vi "StudentDataBase.vi"() -> ()   [LabVIEW 2020]
uses:
  #typedef_Student.ctl
panel:
  out "Repeated students by name":T1[](array[typedef])
  out "Sorted students by number":T1[](array[typedef])
  in  "List of Students":T1[](array[typedef])
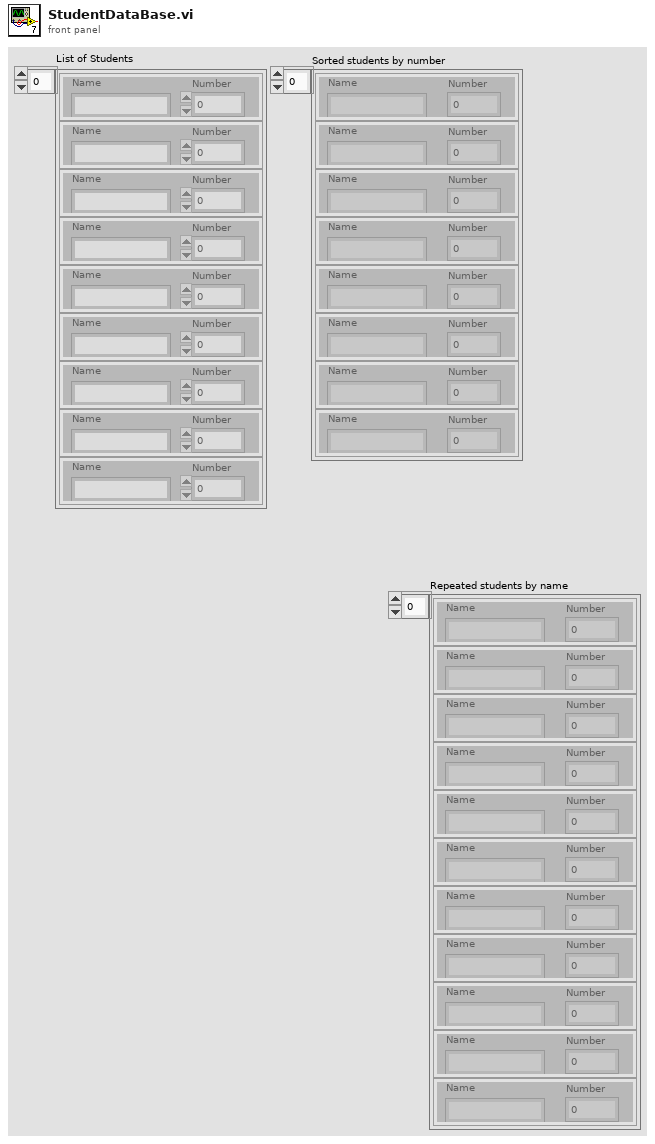
[diagram p1: front panel]
types:
  T1 = typedef "#typedef_Student.ctl" = cluster{"Name":string, "Number":dbl}
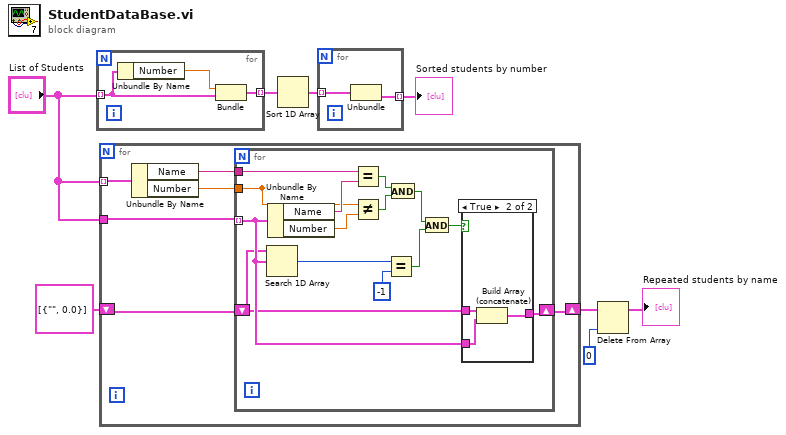
[diagram p0: block diagram]
diagram:
  n1 = for {
    tunnel: "List of Students" -> [w11] mode=indexing
    tunnel: [w9] -> w8 mode=indexing
    n2 = Unbundle By Name(w11) -> ("Number"=w10:dbl)
    n3 = Bundle("Number"=w10, "Students"=w11) -> (w9:cluster{"Number":dbl, "Students":T1})  [unwired: 1 in]
  }
  n4 = for {
    tunnel: "List of Students" -> [w17] mode=indexing
    tunnel: "List of Students" -> [w14]
    shift-right: [w13] -> w3
    shift-left: T1[] [{"Name"="", "Number"=0.0}] -> [w12]
    n5 = Unbundle By Name(w17) -> ("Name"=w16:string, "Number"=w15:dbl)
    n6 = for {
      tunnel: w16 -> [w31]
      tunnel: [w28] -> _ mode=indexing
      tunnel: w15 -> [w28]
      tunnel: w14 -> [w24] mode=indexing
      shift-right: [w25] -> w13
      shift-left: w12 -> [w23]
      n7 = Search 1D Array(1D array=w23, element=w24) -> (index of element=w19:i32)  [unwired: 1 in]
      n8 = Unbundle By Name(w24) -> ("Name"=w30:string, "Number"=w29:dbl)
      n9 = Equal?(x=w31, y=w30) -> (x = y?=w27:bool)
      n10 = Not Equal?(x=w28, y=w29) -> (x != y?=w26:bool)
      n11 = Equal?(x=w19, y=-1) -> (x = y?=w20:bool)
      n12 = And(x=w27, y=w26) -> (x .and. y?=w22:bool)
      n13 = And(x=w22, y=w20) -> (x .and. y?=w21:bool)
      n14 = case shown="True" w21 {
        tunnel: [w32 w34] -> w25
        tunnel: w23 -> [w32 w35]
        tunnel: w24 -> [_ w33]
        frame False {
        }
        frame True {
          n15 = Build Array (concatenate)(w35, w33) -> (w34:T1[])
        }
      }
    }
  }
  n16 = Sort 1D Array(array=w8) -> (sorted array=w7:cluster{"Number":dbl, "Students":T1}[])
  n17 = for {
    tunnel: w7 -> [w37] mode=indexing
    tunnel: [w36] -> w6 mode=indexing
    n18 = Unbundle(w37) -> ("Students"=w36:T1)  [unwired: 1 out]
  }
  "Sorted students by number" <- w6
  n19 = Delete From Array(array=w3, index=0) -> (array with subset deleted=→"Repeated students by name":T1[])  [unwired: 1 in, 1 out]
